vi "Teleop.vi"(10 "Match Info":T1={"Autonomous Elapsed Seconds"=0.0, "TeleOp Elapsed Seconds"=0.0, "Disabled Elapsed Seconds"=0.0, "Visited Autonomous"=FALSE, "Visited TeleOp"=FALSE, "Visited Disabled"=FALSE, "Autonomous Settings"={"Autonomous Style"=enum."Independent", "VI Refnum"=refnum}}, 11 "Call Context":T2) -> ()   [LabVIEW 2019]
doc: "This VI is called for each TeleOp packet received from the DS where the robot is not disabled. It is often used to read from the joysticks and update I/O or to update setpoints for timed control loops. It should complete and return within 20 milliseconds or it may miss DS packets."
uses:
  <vilib>/Rock Robotics/WPI/DriverStation/WPI_DriverStationDerivedRobotMode.ctl
  <vilib>/Rock Robotics/WPI/DriverStation/WPI_DriverStationMatch Info.ctl
  <vilib>/Rock Robotics/WPI/Utilities/WPI_GetSetVariantRefNum.vi
  JoysticksGlobal.vi
  <vilib>/Rock Robotics/Network Tables/NT Read Boolean.vi
  <vilib>/Rock Robotics/Network Tables/NT Read Number.vi
panel:
  out "Sample Slider 0":dbl(slide) scale=0.0..5.0
  out "Sample Boolean 1":bool
  out "Sample Boolean 0":bool
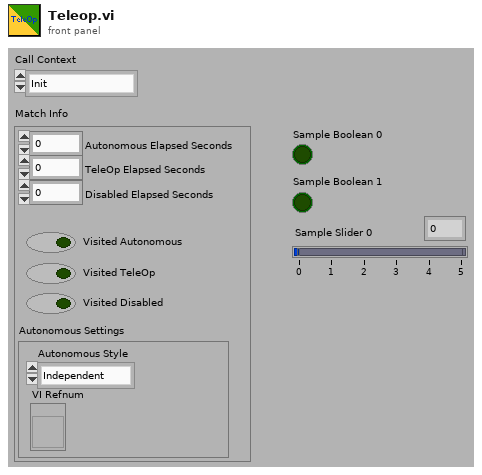
[diagram p1: front panel]
types:
  T1 = typedef "WPI_DriverStationMatch Info.ctl" = cluster{"Autonomous Elapsed Seconds":dbl, "TeleOp Elapsed Seconds":dbl, "Disabled Elapsed Seconds":dbl, "Visited Autonomous":bool, "Visited TeleOp":bool, "Visited Disabled":bool, "Autonomous Settings":cluster{"Autonomous Style":enum16{"Iterative", "Independent"}, "VI Refnum":refnum<vi>}}
  T2 = typedef "WPI_DriverStationDerivedRobotMode.ctl" = enum16{"Init", "Execute", "Stop"}
  T3 = typedef "WPI_JoystickDevRef.ctl" = cluster{"Device":T4}
  T4 = typedef "WPI_JoystickDeviceEnum.ctl" = enum16{"USB 0", "USB 1", "USB 2", "USB 3", "USB 4", "USB 5"}
  T5 = typedef "D-Pad.ctl" = cluster{"Top":bool, "Bottom":bool, "None":bool, "Right":bool, "Left":bool}
  T6 = typedef "Button Cluster.ctl" = cluster{"Buttons[0]":bool, "Buttons[1]":bool, "Buttons[2]":bool, "Buttons[3]":bool, "Buttons[4]":bool, "Buttons[5]":bool, "Buttons[6]":bool, "Buttons[7]":bool, "Buttons[8]":bool, "Buttons[9]":bool}
  T7 = typedef "Axes Cluster.ctl" = cluster{"Axes[0]":dbl, "Axes[1]":dbl, "Axes[2]":dbl, "Axes[3]":dbl, "Axes[4]":dbl, "Axes[5]":dbl, "Axes[6]":dbl, "Axes[7]":dbl, "Axes[8]":dbl}
  T8 = cluster{"Buttons[0]":bool, "Buttons[1]":bool, "Buttons[2]":bool, "Buttons[3]":bool, "Buttons[4]":bool, "Buttons[5]":bool, "Buttons[6]":bool, "Buttons[7]":bool, "Buttons[8]":bool}
  T9 = cluster{"Axes[0]":dbl, "Axes[1]":dbl, "Axes[2]":dbl, "Axes[3]":dbl, "Axes[4]":dbl, "Axes[5]":dbl, "Axes[6]":dbl, "Axes[7]":dbl, "Axes[8]":dbl}
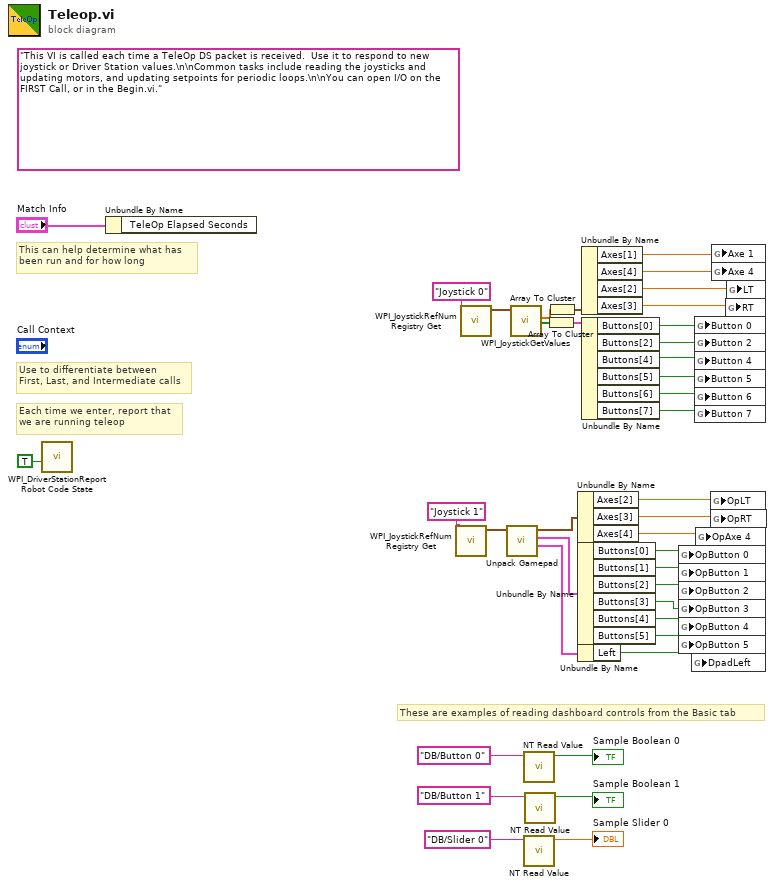
[diagram p0: block diagram]
diagram:
  (unwired) "This VI is called each time a TeleOp DS packet is received.  Use it to respond to new joystick or Driver Station values.\n\nCommon tasks include reading the joysticks and updating motors, and updating setpoints for periodic loops.\n\nYou can open I/O on the FIRST Call, or in the Begin.vi."
  # "These are examples of reading dashboard controls from the Basic tab"
  # "Each time we enter, report that\nwe are running teleop"
  # "Use to differentiate between\nFirst, Last, and Intermediate calls"
  # "This can help determine what has\nbeen run and for how long"
  n1 = call <vilib>:"WPI_DriverStationReport Robot Code State.vi"("TeleOp"=TRUE ("Autonomous")) -> ()  [unwired: 10 in, 1 out]
  n2 = Unbundle By Name("Match Info") -> ()  [unwired: 1 out]
  n3 = call <vilib>:"WPI_JoystickRefNum Registry Get.vi"("refnum name"="Joystick 1") -> ("JoystickDevRef"=w20:T3)  [unwired: 1 in, 9 out]
  n4 = call <vilib>:"WPI_JoystickRefNum Registry Get.vi"("refnum name"="Joystick 0") -> ("JoystickDevRef"=w37:T3)  [unwired: 1 in, 9 out]
  n5 = call "Unpack Gamepad.vi"("JoystickDevRef"=w20) -> ("D-Pad"=w18:T5, "Button Cluster"=w19:T6, "Axes"=w10:T7)  [unwired: 8 in]
  n6 = call <vilib>:"WPI_JoystickGetValues.vi"("JoystickDevRef"=w37) -> ("Buttons"=w29:bool[], "Axes"=w24:dbl[])  [unwired: 6 in, 3 out]
  n7 = call-poly <vilib>:"NT Read Value.vi"("Name"="DB/Button 0" ("refnum name")) -> ("Boolean"=→"Sample Boolean 0":bool)  [unwired: 9 in, 1 out]
  n8 = call-poly <vilib>:"NT Read Value.vi"("Name"="DB/Slider 0" ("refnum name")) -> ("Numeric"=→"Sample Slider 0":dbl)  [unwired: 9 in, 1 out]
  n9 = call-poly <vilib>:"NT Read Value.vi"("Name"="DB/Button 1" ("refnum name")) -> ("Boolean"=→"Sample Boolean 1":bool)  [unwired: 9 in, 1 out]
  n10 = Array To Cluster(array=w29) -> (cluster=w28:T8)
  n11 = Array To Cluster(array=w24) -> (cluster=w25:T9)
  n12 = Unbundle By Name(w10) -> ("Axes[2]"=w9:dbl, "Axes[3]"=w8:dbl, "Axes[4]"=w7:dbl)
  n13 = Unbundle By Name(w19) -> ("Buttons[0]"=w17:bool, "Buttons[1]"=w16:bool, "Buttons[2]"=w15:bool, "Buttons[3]"=w11:bool, "Buttons[4]"=w12:bool, "Buttons[5]"=w13:bool)
  n14 = Unbundle By Name(w18) -> ("Left"=w14:bool)
  n15 = Unbundle By Name(w25) -> ("Axes[1]"=w23:dbl, "Axes[4]"=w22:dbl, "Axes[2]"=w2:dbl, "Axes[3]"=w1:dbl)
  n16 = Unbundle By Name(w28) -> ("Buttons[0]"=w4:bool, "Buttons[2]"=w3:bool, "Buttons[4]"=w26:bool, "Buttons[5]"=w27:bool, "Buttons[6]"=w5:bool, "Buttons[7]"=w6:bool)
  n17 = global write "JoysticksGlobal.vi" "OpButton 0"(w17) -> ()
  n18 = global write "JoysticksGlobal.vi" "OpButton 1"(w16) -> ()
  n19 = global write "JoysticksGlobal.vi" "OpButton 2"(w15) -> ()
  n20 = global write "JoysticksGlobal.vi" "OpButton 3"(w11) -> ()
  n21 = global write "JoysticksGlobal.vi" "OpButton 4"(w12) -> ()
  n22 = global write "JoysticksGlobal.vi" "OpButton 5"(w13) -> ()
  n23 = global write "JoysticksGlobal.vi" "DpadLeft"(w14) -> ()
  n24 = global write "JoysticksGlobal.vi" "Button 0"(w4) -> ()
  n25 = global write "JoysticksGlobal.vi" "Button 2"(w3) -> ()
  n26 = global write "JoysticksGlobal.vi" "Button 4"(w26) -> ()
  n27 = global write "JoysticksGlobal.vi" "Button 5"(w27) -> ()
  n28 = global write "JoysticksGlobal.vi" "Button 6"(w5) -> ()
  n29 = global write "JoysticksGlobal.vi" "Button 7"(w6) -> ()
  n30 = global write "JoysticksGlobal.vi" "OpAxe 4"(w7) -> ()
  n31 = global write "JoysticksGlobal.vi" "OpLT"(w9) -> ()
  n32 = global write "JoysticksGlobal.vi" "OpRT"(w8) -> ()
  n33 = global write "JoysticksGlobal.vi" "Axe 1"(w23) -> ()
  n34 = global write "JoysticksGlobal.vi" "Axe 4"(w22) -> ()
  n35 = global write "JoysticksGlobal.vi" "RT"(w1) -> ()
  n36 = global write "JoysticksGlobal.vi" "LT"(w2) -> ()
